vi "WakeOnLan.vi"(7 "port":u16=7, 8 "error in (no error)":errorcluster, 9 "local port":u16, 10 "MAC-address":string="\u0000€/!zð", 11 "IP-address":string="192.168.150.78") -> (0 "error out":errorcluster)   [LabVIEW 2015]
doc: "Dieses VI sendet ein \"magic packet\", um den PC mit der gewünschten MAC-Adresse via Power on LAN zu starten. Das \"magic packet wird via UDP an die angegebene Netzwerkadresse gesendet. Ist keine Netzwerkadresse angegeben oder die Netzwerkadresse ungültig, so wird das \"magic packet\" über die Broadcast-Adresse des gesamten Netzes versandt"
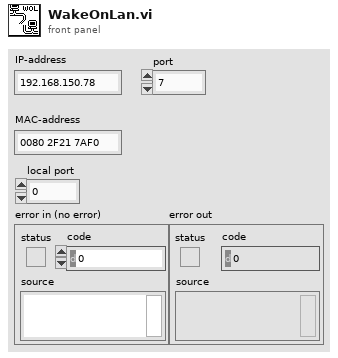
[diagram p1: front panel]
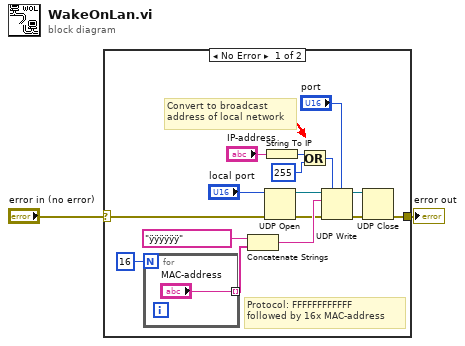
[diagram p0: block diagram]
diagram:
  n1 = case shown="No Error" "error in (no error)" {
    selector: "error in (no error)" -> [w10 w20]
    tunnel: [w9 w20] -> w1
    frame No Error {
      # "Convert to broadcast\naddress of local network"
      # "Protocol: FFFFFFFFFFFF\nfollowed by 16x MAC-address"
      n2 = for {
        N: 16 -> [_]
        tunnel: ["MAC-address"] -> w13 mode=indexing
      }
      n3 = Concatenate Strings("ÿÿÿÿÿÿ", w13) -> (w12:string)
      n4 = UDP Open(8:w10, 11:"local port") -> (port=w18:refnum<k16>, 0:w11:errorcluster)  [unwired: 3 in, 1 out]
      n5 = String To IP(1:"IP-address") -> (0:w6:u32)
      n6 = Or(x=w6, y=u32 255) -> (x .or. y?=w7:u32)
      n7 = UDP Write(address=w7, port or service name="port", connection ID=w18, data in=w12, 8:w11) -> (error out=w17:errorcluster, 3:w16:refnum<k16>)  [unwired: 1 in]
      n8 = UDP Close(connection ID=w16, 8:w17) -> (error out=w9:errorcluster)  [unwired: 1 out]
    }
    frame Error {
    }
  }
  "error out" <- w1
